vi "Set AO sync.vi"(8 "error in":errorcluster, 9 "AO sync":bool, 11 "FPGA SPI config ref":T1) -> (0 "error out":errorcluster, 3 "FPGA SPI config out":T1)   [LabVIEW 2013]
uses:
  FPGA_spi_config.ctl
  <vilib>/rvi/interface/common/niFpgaWaitOnOcc.vi
  <vilib>/Utility/error.llb/Error Cluster From Error Code.vi
  <vilib>/rvi/errors/niLvFpgaAdjustHostInterfaceError.vi
  <vilib>/rvi/interface/nirviReadWriteControl/nirviReadWriteControl.xnode
  NiFpgaLv.dll
  <vilib>/rvi/interface/Simulation/niFpgaSimulationCallBeginRW.vi
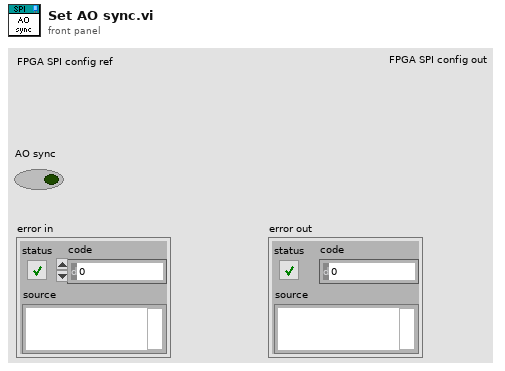
[diagram p1: front panel]
types:
  T1 = typedef "FPGA_spi_config.ctl" = refnum<k20>
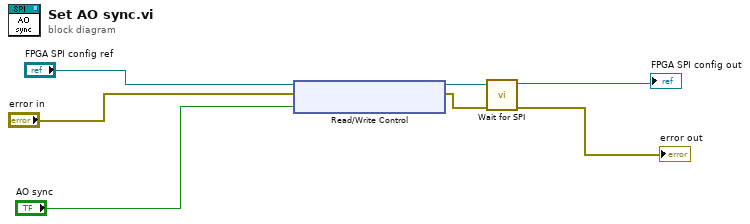
[diagram p0: block diagram]
diagram:
  n1 = xnode "Read/Write Control"("FPGA VI Reference In"="FPGA SPI config ref", "error in"="error in", "IO Module\\AO Data Sync"="AO sync") -> ("FPGA VI Reference Out"=w4:T1, "error out"=w2:errorcluster)
  n2 = call "Wait for SPI.vi"("error in"=w2, "FPGA SPI config ref"=w4) -> ("error out"=→"error out":errorcluster, "FPGA SPI config out"=→"FPGA SPI config out":T1)  [unwired: 7 in, 1 out]
